vi "Read Analog Output Parameters.vi"(8 "error in (no error)":errorcluster, 11 "Analog_Output in":refnum<class "Analog_Output.lvclass">) -> (0 "error out":errorcluster, 2 "Analog Output Parameters":T1={"Enable Analog Out?"=FALSE, "Physical Channel"="PXI1Slot2/ao0:2", "Minimum Value"=-10.0, "Maximum Value"=10.0, "Samples per second"=0.0, "Total AO Time (seconds)"=0.0, "Start Trigger"={"Wait for start trigger?"=FALSE, "source"="/Dev1/PFI0", "edge"=10280}, "Analog Output Waveforms (channel, time)"=[], "Export trigger"={"Export Start Trigger?"=FALSE, "output terminal"=""}} {"Start Trigger"."edge" items=["Rising"=10280, "Falling"=10171]; "Maximum Value" format="%0.2f"; "Minimum Value" format="%0.2f"}, 3 "Analog_Output out":refnum<class "Analog_Output.lvclass">)   [LabVIEW 2013, in "Analog_Output.lvclass"]
uses:
  Analog_Output.lvclass
  AO_settings.ctl
  Analog_Output.lvclass/Analog_Output.ctl
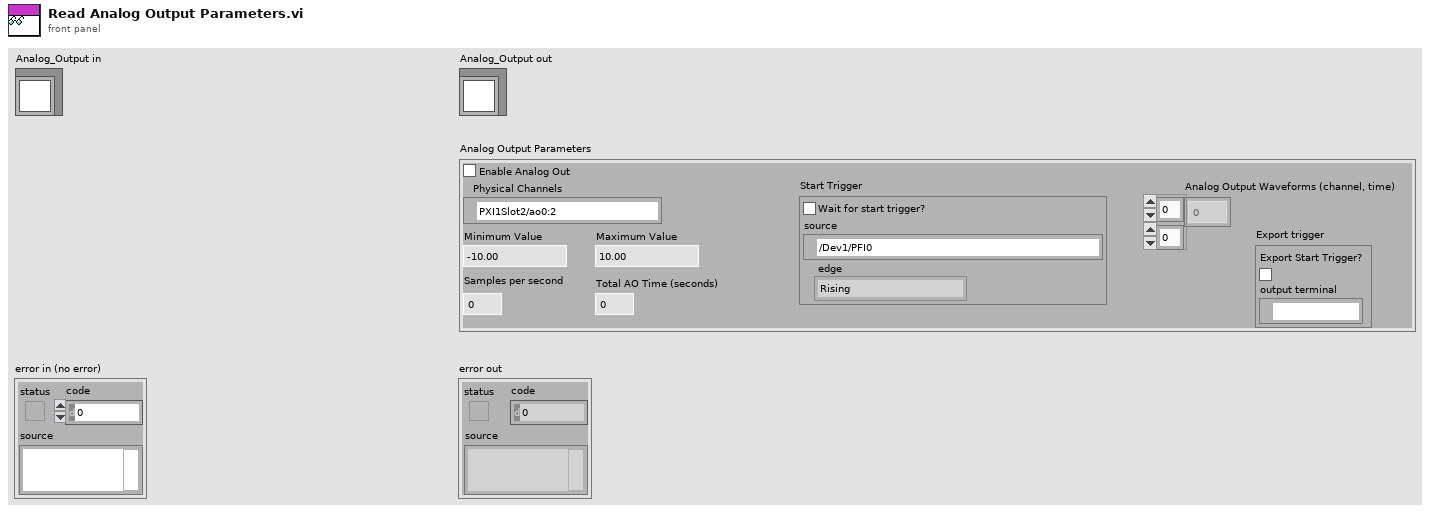
[diagram p1: front panel]
types:
  T1 = typedef "Analog_Output.lvclass/AO_settings.ctl" = cluster{"Enable Analog Out?":bool, "Physical Channel":tag, "Minimum Value":dbl, "Maximum Value":dbl, "Samples per second":dbl, "Total AO Time (seconds)":dbl, "Start Trigger":cluster{"Wait for start trigger?":bool, "source":tag, "edge":i32}, "Analog Output Waveforms (channel, time)":dbl[][], "Export trigger":cluster{"Export Start Trigger?":bool, "output terminal":tag}}
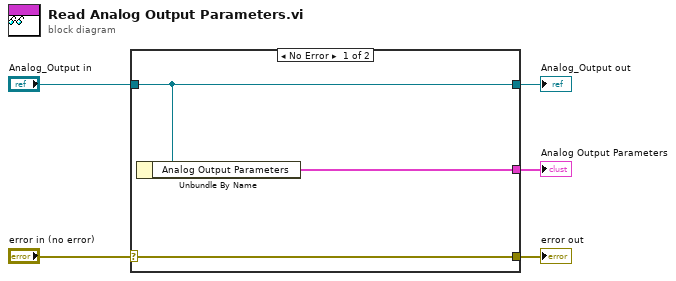
[diagram p0: block diagram]
diagram:
  n1 = case shown="No Error" "error in (no error)" {
    selector: "error in (no error)" -> [w8 w9]
    tunnel: [w8 w9] -> w4
    tunnel: [w7 w10] -> w2
    tunnel: "Analog_Output in" -> [w7 w10]
    tunnel: [w6 _] -> w1
    frame No Error {
      n2 = Unbundle By Name(w7) -> ("Analog Output Parameters"=w6:T1)
    }
    frame Error {
    }
  }
  "error out" <- w4
  "Analog_Output out" <- w2
  "Analog Output Parameters" <- w1
